vi "Validate Test Vector.vi"(8 "error in (no error)":errorcluster, 11 "LUnit Test Vector in":refnum<class "LUnit Test Vector.lvclass">) -> (0 "error out":errorcluster, 2 "Valid?":bool, 3 "LUnit Test Vector out":refnum<class "LUnit Test Vector.lvclass">)   [LabVIEW 2020, in "LUnit Test Vector.lvclass"]
uses:
  LUnit Test Vector.lvclass
  Test Case/LUnit Test Case.lvclass
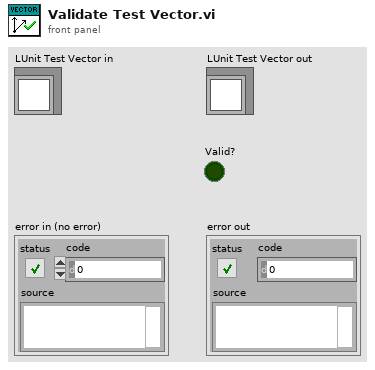
[diagram p1: front panel]
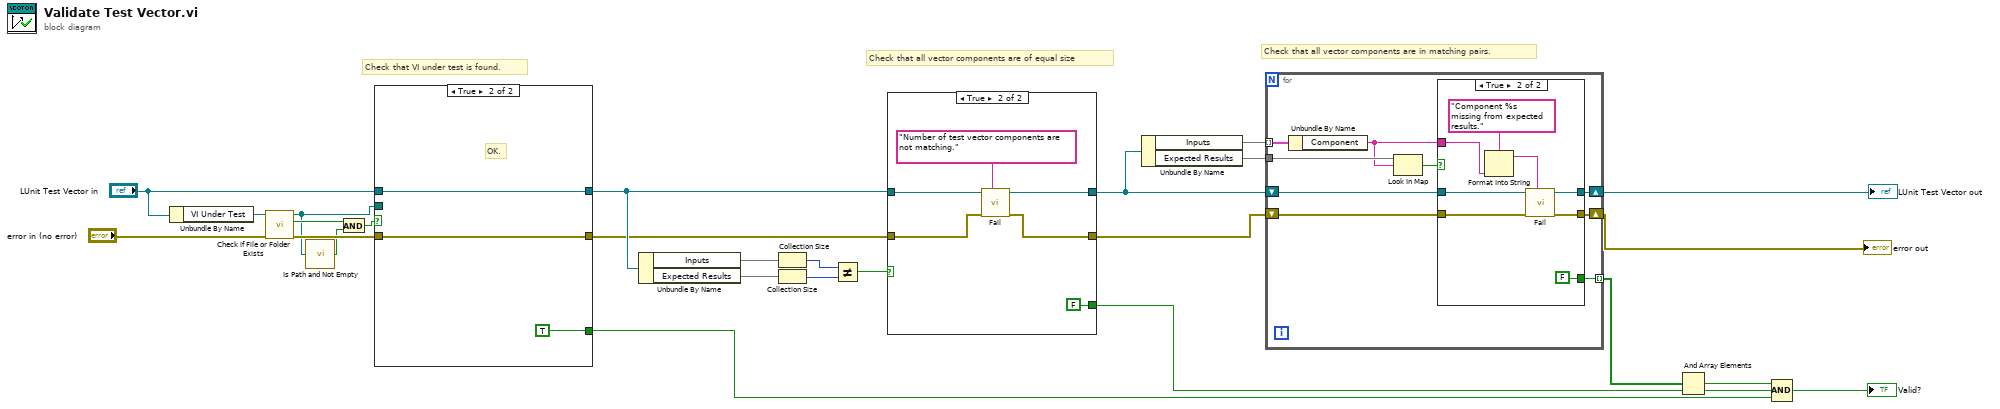
[diagram p0: block diagram]
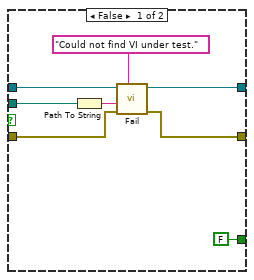
[diagram p2: hidden frame]
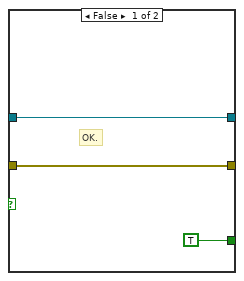
[diagram p3: hidden frame]
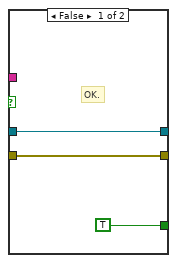
[diagram p4: hidden frame]
diagram:
  # "Check that VI under test is found."
  # "Check that all vector components are in matching pairs."
  # "Check that all vector components are of equal size"
  n1 = Unbundle By Name("LUnit Test Vector in") -> ("VI Under Test"=w15:path)
  n2 = call <vilib>:"Check if File or Folder Exists.vi"("error in (no error)"="error in (no error)", "path"=w15) -> ("error out"=w10:errorcluster, "file or folder exists?"=w13:bool, "dup path"=w2:path)  [unwired: 7 in]
  n3 = call <vilib>:"Is Path and Not Empty.vi"("path"=w2) -> ("Is Path and Not Empty?"=w1:bool)  [unwired: 4 in]
  n4 = And(x=w13, y=w1) -> (x .and. y?=w3:bool)
  n5 = case shown="True" w3 {
    tunnel: "LUnit Test Vector in" -> [w34 w37]
    tunnel: [w33 w37] -> w11
    tunnel: w10 -> [w32 w36]
    tunnel: [w31 w36] -> w9
    tunnel: w2 -> [w28 _]
    tunnel: [FALSE TRUE] -> w6
    frame False {
      n6 = Path To String(path=w28) -> (string=w29:string)
      n7 = call "Fail.vi"("Description"="Could not find VI under test.", "error in (no error)"=w32, "Message"=w29, "LUnit Test Case In"=w34) -> ("error out"=w31:errorcluster, "LUnit Test Case Out"=w33:refnum<class "LUnit Test Vector.lvclass">)  [unwired: 6 in]
    }
    frame True {
      # "OK."
    }
  }
  n8 = Unbundle By Name(w11) -> ("Inputs"=w26:map{string, map{string, variant}}, "Expected Results"=w25:map{string, map{string, variant}})
  n9 = Collection Size(1:w26) -> (0:w24:i32)
  n10 = Collection Size(1:w25) -> (0:w23:i32)
  n11 = Not Equal?(x=w24, y=w23) -> (x != y?=w22:bool)
  n12 = case shown="True" w22 {
    tunnel: [w40 w46] -> w18
    tunnel: w9 -> [w40 w45]
    tunnel: [w39 w44] -> w19
    tunnel: w11 -> [w39 w43]
    tunnel: [TRUE FALSE] -> w7
    frame False {
      # "OK."
    }
    frame True {
      n13 = call "Fail.vi"("Description"="Number of test vector components are not matching.", "error in (no error)"=w45, "LUnit Test Case In"=w43) -> ("error out"=w46:errorcluster, "LUnit Test Case Out"=w44:refnum<class "LUnit Test Vector.lvclass">)  [unwired: 7 in]
    }
  }
  n14 = Unbundle By Name(w19) -> ("Inputs"=w21:map{string, map{string, variant}}, "Expected Results"=w20:map{string, map{string, variant}})
  n15 = for {
    tunnel: w21 -> [w55] mode=indexing
    tunnel: w20 -> [w54]
    shift-right: [w51] -> w16
    shift-left: w19 -> [w52]
    shift-right: [w49] -> w17
    shift-left: w18 -> [w50]
    tunnel: [w47] -> w8 mode=indexing
    n16 = Unbundle By Name(w55) -> ("Component"=w48:string)
    n17 = Look In Map(map=w54, key=w48) -> (key not found?=w53:bool)  [unwired: 1 in, 1 out]
    n18 = case shown="True" w53 {
      tunnel: w52 -> [w57 w66]
      tunnel: [w57 w65] -> w51
      tunnel: w50 -> [w58 w64]
      tunnel: [w58 w63] -> w49
      tunnel: w48 -> [_ w61]
      tunnel: [TRUE FALSE] -> w47
      frame False {
        # "OK."
      }
      frame True {
        n19 = Format Into String(format string="Component %s missing from expected results.", w61) -> (resulting string=w60:string)  [unwired: 2 in, 1 out]
        n20 = call "Fail.vi"("Description"=w60, "error in (no error)"=w64, "LUnit Test Case In"=w66) -> ("error out"=w63:errorcluster, "LUnit Test Case Out"=w65:refnum<class "LUnit Test Vector.lvclass">)  [unwired: 7 in]
      }
    }
  }
  "error out" <- w17
  "LUnit Test Vector out" <- w16
  n21 = And Array Elements(Boolean array=w8) -> (logical AND=w5:bool)
  n22 = Compound Arithmetic op=AND(w5, w7, w6) -> (→"Valid?":bool)
